vi "Refresh Data to Listbox Format.vi"(8 "error in":errorcluster, 10 "Refresh Port":T1[](array[typedef])) -> (0 "error out":errorcluster, 2 "Refresh Listbox":T5)   [LabVIEW 2020, in "Communication Bus Template System Explorer.lvlib" / "Implementation.lvlib"]
uses:
  Implementation.lvlib
  Types/Refresh Listbox.ctl
  Types/Refresh Symbols.ctl
  Types/Refresh Port.ctl
  Types/Refresh Frame.ctl
  Types/Refresh Signal.ctl
  Types/ECU.ctl
  <vilib>/NI VeriStand/Custom Device API/Custom Device Channel Type.ctl
  <vilib>/NI VeriStand/Custom Device API/Custom Device API.lvlib
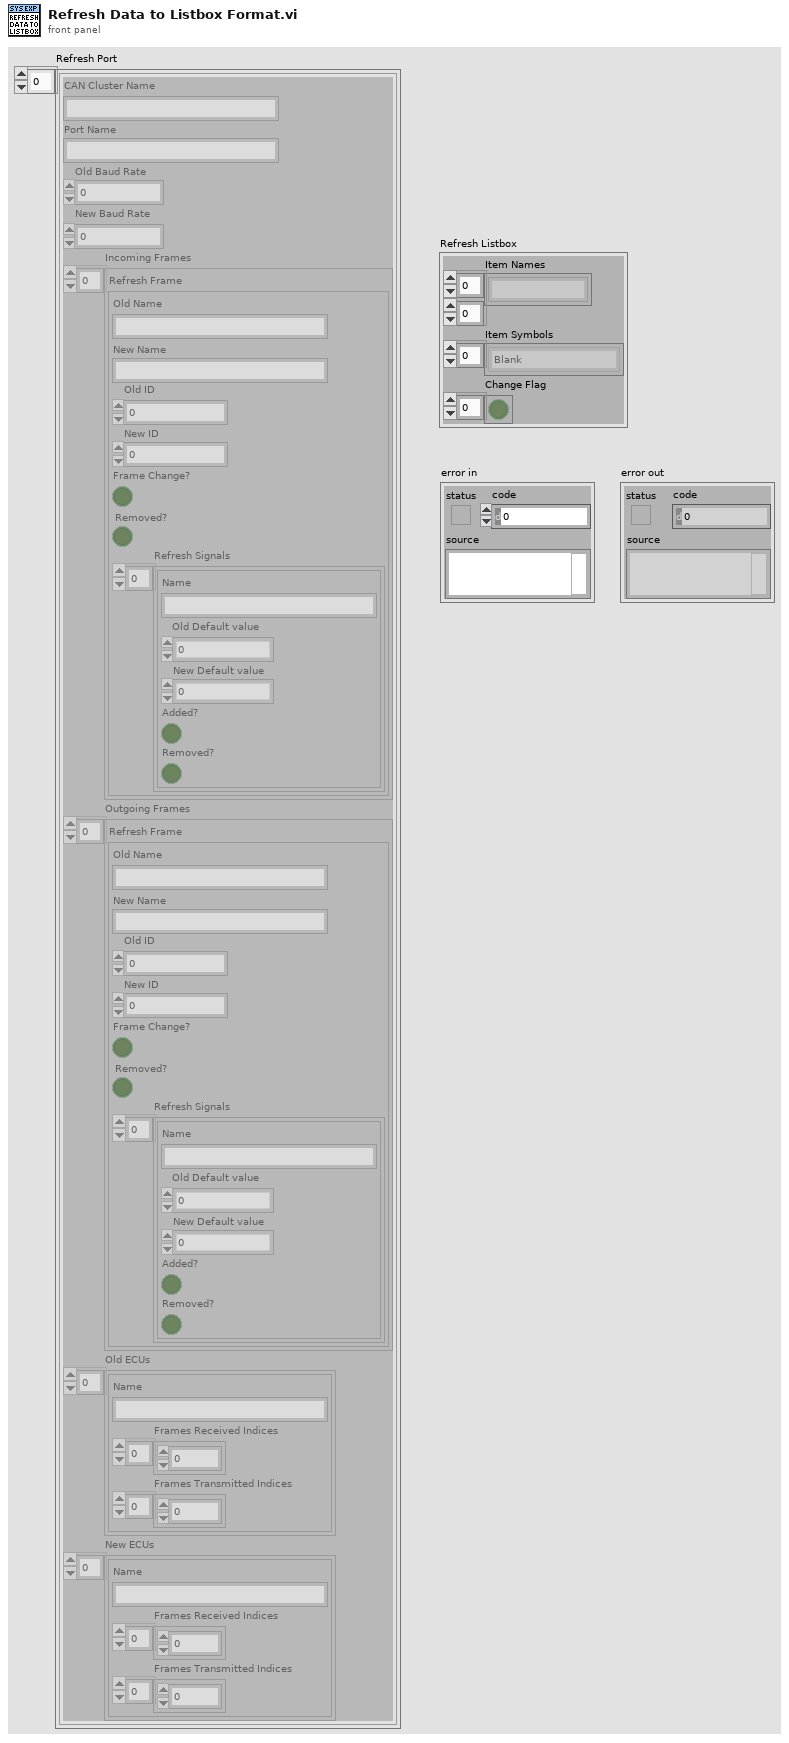
[diagram p1: front panel]
types:
  T1 = typedef "Communication Bus Template System Explorer.lvlib/Implementation.lvlib/Refresh Port.ctl" = cluster{"CAN Cluster Name":string, "Port Name":string, "Old Baud Rate":u64, "New Baud Rate":u64, "Incoming Frames":T2[], "Outgoing Frames":T2[], "Old ECUs":T4[], "New ECUs":T4[]}
  T2 = typedef "Communication Bus Template System Explorer.lvlib/Implementation.lvlib/Refresh Frame.ctl" = cluster{"Old Name":string, "New Name":string, "Old ID":u32, "New ID":u32, "Frame Change?":bool, "Removed?":bool, "Refresh Signals":T3[]}
  T3 = typedef "Communication Bus Template System Explorer.lvlib/Implementation.lvlib/Refresh Signal.ctl" = cluster{"Name":string, "Old Default value":dbl, "New Default value":dbl, "Added?":bool, "Removed?":bool}
  T4 = typedef "Communication Bus Template System Explorer.lvlib/Implementation.lvlib/ECU.ctl" = cluster{"Name":string, "Frames Received Indices":u32[], "Frames Transmitted Indices":u32[]}
  T5 = typedef "Communication Bus Template System Explorer.lvlib/Implementation.lvlib/Refresh Listbox.ctl" = cluster{"Item Names":string[][], "Item Symbols":T6[], "Change Flag":bool[]}
  T6 = typedef "Communication Bus Template System Explorer.lvlib/Implementation.lvlib/Refresh Symbols.ctl" = enum16{"Blank", "Port", "Incoming", "Outgoing", "Frame", "Signal", "Cluster", "Baud Rate"}
  T7 = typedef "Custom Device API.lvlib/Custom Device Channel Type.ctl" = enum16{"Input", "Output"}
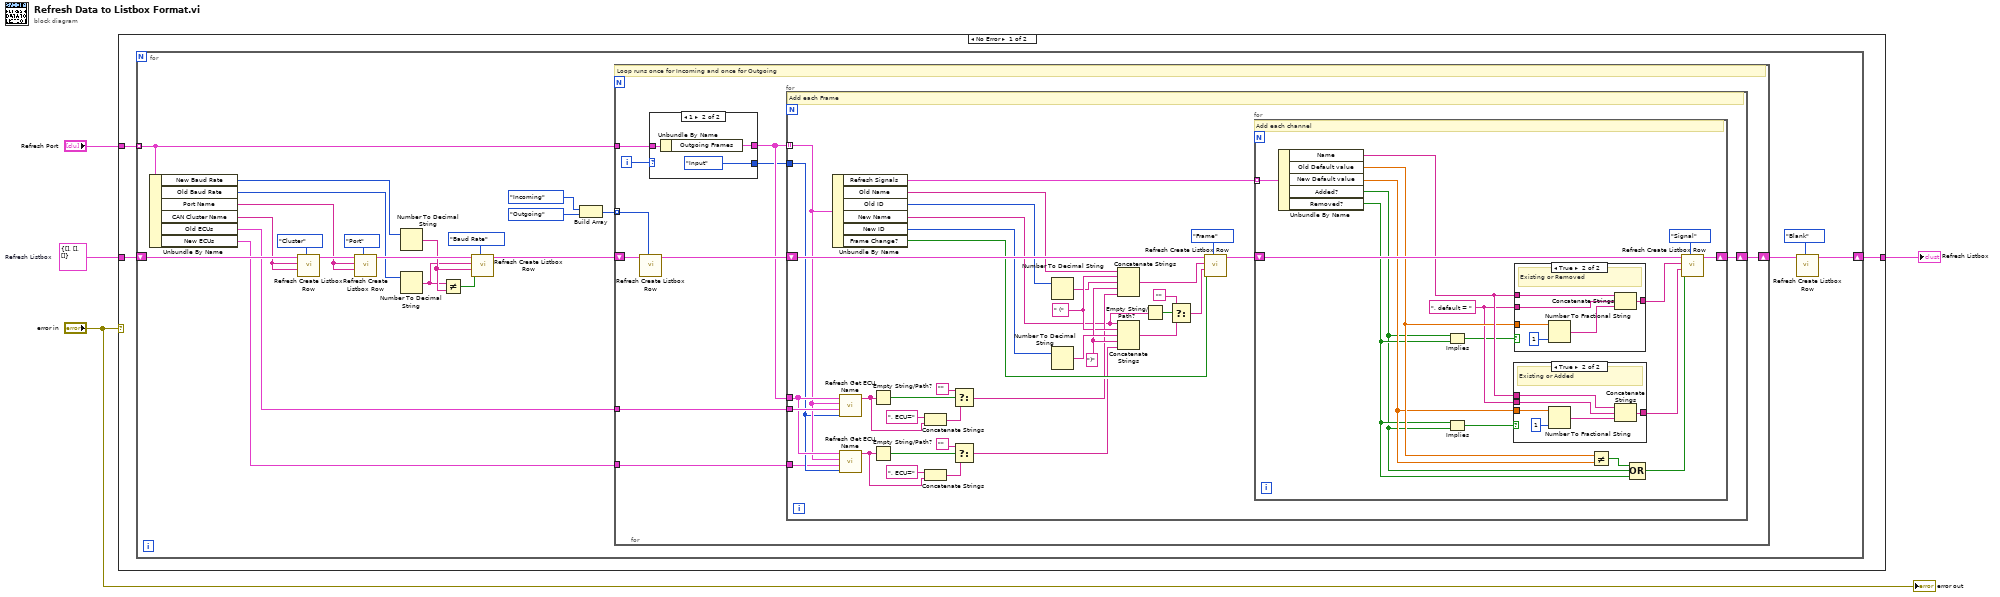
[diagram p0: block diagram]
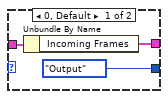
[diagram p2: hidden frame]
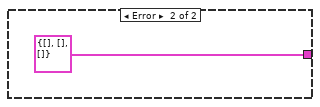
[diagram p5: hidden frame]
diagram:
  w2 = T5 {"Item Names"=[], "Item Symbols"=[], "Change Flag"=[]}  # Refresh Listbox
  n1 = case shown="No Error" "error in" {
    tunnel: [w5 T5 {"Item Names"=[], "Item Symbols"=[], "Change Flag"=[]} ("Refresh Listbox out")] -> w1
    tunnel: w2 -> [w7 _]
    tunnel: "Refresh Port" -> [w6 _]
    frame No Error {
      n2 = for {
        tunnel: w6 -> [w14] mode=indexing
        shift-right: [w11] -> w5
        shift-left: w7 -> [w20]
        n3 = Unbundle By Name(w14) -> ("New Baud Rate"=w16:u64, "Old Baud Rate"=w15:u64, "Port Name"=w17:string, "CAN Cluster Name"=w18:string, "Old ECUs"=w9:T4[], "New ECUs"=w8:T4[])
        n4 = call "Refresh Create Listbox Row.vi"("Refresh Symbol (Blank)"=Refresh_Symbols."Cluster" ("Refresh Symbols"), "New Item"=w18, "Old Item"=w18, "Refresh Listbox"=w20) -> ("Refresh Listbox out"=w19:T5)  [unwired: 7 in]
        n5 = call "Refresh Create Listbox Row.vi"("Refresh Symbol (Blank)"=Refresh_Symbols."Port" ("Refresh Symbols"), "New Item"=w17, "Old Item"=w17, "Refresh Listbox"=w19) -> ("Refresh Listbox out"=w24:T5)  [unwired: 7 in]
        n6 = Number To Decimal String(number=w16) -> (decimal integer string=w23:string)  [unwired: 1 in]
        n7 = Number To Decimal String(number=w15) -> (decimal integer string=w21:string)  [unwired: 1 in]
        n8 = Not Equal?(x=w21, y=w23) -> (x != y?=w22:bool)
        n9 = call "Refresh Create Listbox Row.vi"("Refresh Symbol (Blank)"=Refresh_Symbols."Baud Rate" ("Refresh Symbols"), "Change? (T)"=w22, "New Item"=w23, "Old Item"=w21, "Refresh Listbox"=w24) -> ("Refresh Listbox out"=w29:T5)  [unwired: 6 in]
        n10 = Build Array(Refresh_Symbols."Incoming" ("Refresh Symbols"), Refresh_Symbols."Outgoing" ("Refresh Symbols")) -> (w26:T6[])
        n11 = for {
          shift-right: [w37] -> w12
          shift-left: w29 -> [w40]
          tunnel: w26 -> [w39] mode=indexing
          tunnel: w14 -> [w35]
          tunnel: w9 -> [w33]
          tunnel: w8 -> [w31]
          i -> [w36]
          # "Loop runs once for Incoming and once for Outgoing"
          n12 = call "Refresh Create Listbox Row.vi"("Refresh Symbol (Blank)"=w39, "Refresh Listbox"=w40) -> ("Refresh Listbox out"=w38:T5)  [unwired: 9 in]
          n13 = case shown="1" w36 {
            tunnel: [w42 w46] -> w34
            tunnel: w35 -> [w43 w45]
            tunnel: [Custom_Device_Channel_Type."Output" ("Type (Input)") Custom_Device_Channel_Type."Input" ("Type (Input)")] -> w32
            frame 0, Default {
              n14 = Unbundle By Name(w43) -> ("Incoming Frames"=w42:T2[])
            }
            frame 1 {
              n15 = Unbundle By Name(w45) -> ("Outgoing Frames"=w46:T2[])
            }
          }
          n16 = for {
            shift-right: [w70] -> w37
            shift-left: w38 -> [w82]
            tunnel: w34 -> [w66] mode=indexing
            tunnel: w34 -> [w67]
            tunnel: w33 -> [w68]
            tunnel: w32 -> [w65]
            tunnel: w31 -> [w64]
            w78 = ")" ("string")
            w77 = " ("
            # "Add each Frame"
            n17 = Unbundle By Name(w66) -> ("Refresh Signals"=w69:T3[], "Old Name"=w74:string, "Old ID"=w73:u32, "New Name"=w51:string, "New ID"=w72:u32, "Frame Change?"=w71:bool)
            n18 = call "Refresh Get ECU Name.vi"("Type (Input)"=w65, "ECUs"=w68, "Refresh Frame"=w66, "Frames"=w67) -> ("ECU Name"=w60:string)  [unwired: 7 in]
            n19 = call "Refresh Get ECU Name.vi"("Type (Input)"=w65, "ECUs"=w64, "Refresh Frame"=w66, "Frames"=w67) -> ("ECU Name"=w53:string)  [unwired: 7 in]
            n20 = Empty String/Path?(string/path=w60) -> (empty?=w62:bool)
            n21 = Empty String/Path?(string/path=w53) -> (empty?=w55:bool)
            n22 = Concatenate Strings(", ECU=", w60) -> (w59:string)
            n23 = Concatenate Strings(", ECU=", w53) -> (w57:string)
            n24 = Select(t="", s=w62, f=w59) -> (s? t:f=w58:string)
            n25 = Select(t="", s=w55, f=w57) -> (s? t:f=w52:string)
            n26 = Number To Decimal String(number=w73) -> (decimal integer string=w76:string)  [unwired: 1 in]
            n27 = Number To Decimal String(number=w72) -> (decimal integer string=w80:string)  [unwired: 1 in]
            n28 = Concatenate Strings(w74, w77, w76, w78, w58) -> (w75:string)
            n29 = Concatenate Strings(w51, w77, w80, w78, w52) -> (w49:string)
            n30 = Empty String/Path?(string/path=w51) -> (empty?=w50:bool)
            n31 = Select(t="", s=w50, f=w49) -> (s? t:f=w48:string)
            n32 = call "Refresh Create Listbox Row.vi"("Refresh Symbol (Blank)"=Refresh_Symbols."Frame", "Change? (T)"=w71, "New Item"=w48, "Old Item"=w75, "Refresh Listbox"=w82) -> ("Refresh Listbox out"=w81:T5)  [unwired: 6 in]
            n33 = for {
              shift-right: [w97] -> w70
              shift-left: w81 -> [w98]
              tunnel: w69 -> [w96] mode=indexing
              w87 = ", default = "
              # "Add each channel"
              n34 = Unbundle By Name(w96) -> ("Name"=w95:string, "Old Default value"=w94:dbl, "New Default value"=w90:dbl, "Added?"=w83:bool, "Removed?"=w84:bool)
              n35 = Implies(1:w84, 2:w83) -> (0:w85:bool)
              n36 = Implies(1:w83, 2:w84) -> (0:w86:bool)
              n37 = case shown="True" w86 {
                tunnel: w95 -> [_ w104]
                tunnel: [_ w102] -> w91
                tunnel: w90 -> [_ w101]
                tunnel: w87 -> [_ w100]
                frame False {
                }
                frame True {
                  # "Existing or Added"
                  n38 = Number To Fractional String(number=w101, precision (6)=i16 1) -> (F-format string=w103:string)  [unwired: 2 in]
                  n39 = Concatenate Strings(w104, w100, w103) -> (w102:string)
                }
              }
              n40 = case shown="True" w85 {
                tunnel: w95 -> [_ w110]
                tunnel: w94 -> [_ w109]
                tunnel: w87 -> [_ w107]
                tunnel: [_ w106] -> w92
                frame False {
                }
                frame True {
                  # "Existing or Removed"
                  n41 = Number To Fractional String(number=w109, precision (6)=i16 1) -> (F-format string=w108:string)  [unwired: 2 in]
                  n42 = Concatenate Strings(w110, w107, w108) -> (w106:string)
                }
              }
              n43 = Not Equal?(x=w94, y=w90) -> (x != y?=w88:bool)
              n44 = Compound Arithmetic op=OR(w88, w83, w84) -> (w89:bool)
              n45 = call "Refresh Create Listbox Row.vi"("Refresh Symbol (Blank)"=Refresh_Symbols."Signal", "Change? (T)"=w89, "New Item"=w91, "Old Item"=w92, "Refresh Listbox"=w98) -> ("Refresh Listbox out"=w97:T5)  [unwired: 6 in]
            }
          }
        }
        n46 = call "Refresh Create Listbox Row.vi"("Refresh Symbol (Blank)"=Refresh_Symbols."Blank", "Refresh Listbox"=w12) -> ("Refresh Listbox out"=w11:T5)  [unwired: 9 in]
      }
    }
    frame Error {
    }
  }
  "Refresh Listbox" <- w1
  "error out" <- "error in"
